vi "(백업)update setup complete.vi"   [LabVIEW 2014]
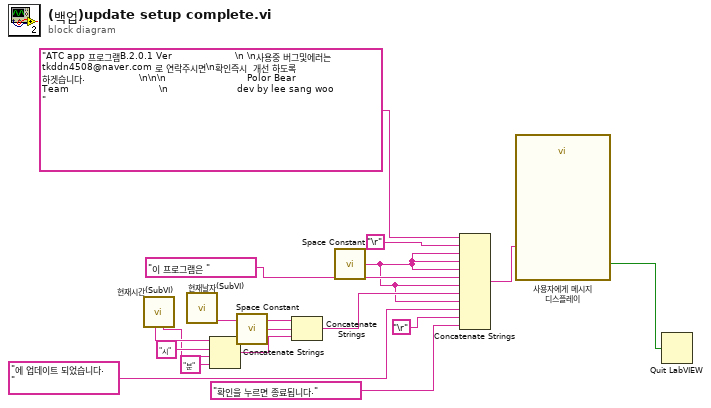
[diagram p0: block diagram]
diagram:
  n1 = call "현재시간(SubVI).vi"() -> ("분 문자열"=w14:string, "시 문자열"=w16:string)  [unwired: 3 in, 7 out]
  n2 = call "현재날자(SubVI).vi"() -> ("월,일 을 문자열로"=w10:string)  [unwired: 5 in, 6 out]
  n3 = Concatenate Strings(w16, "시", w14, "분" ("문자열")) -> (w12:string)
  n4 = call <vilib>:"Space Constant.vi"() -> ("String"=w11:string)
  n5 = Concatenate Strings(w10, w11, w12) -> (w5:string)
  n6 = call <vilib>:"Space Constant.vi"() -> ("String"=w4:string)
  n7 = Concatenate Strings("ATC app 프로그램B.2.0.1 Ver                     \n \n사용중 버그및에러는 tkddn4508@naver.com 로 연락주시면\n확인즉시  개선 하도록 하겟습니다.                  \n\n\n                           Polor Bear Team                              \n                       dev by lee sang woo                            " ("Message"), "\r", w4, w4, w4, "이 프로그램은 ", w4, w5, w4, "에 업데이트 되었습니다.", "\r", "확인을 누르면 종료됩니다.") -> (w17:string)
  n8 = call "사용자에게 메시지 디스플레이"("Message"=w17) -> ("닫기"=w9:bool)  [unwired: 9 in, 1 out]
  n9 = Quit LabVIEW(quit? (T)=w9) -> ()
